vi "destroy.vi"(8 "error in":errorcluster, 11 "queue reporter in":refnum<class "queue reporter.lvclass">) -> (0 "error out":errorcluster)   [LabVIEW 2013, in "queue reporter.lvclass"]
uses:
  queue reporter.lvclass
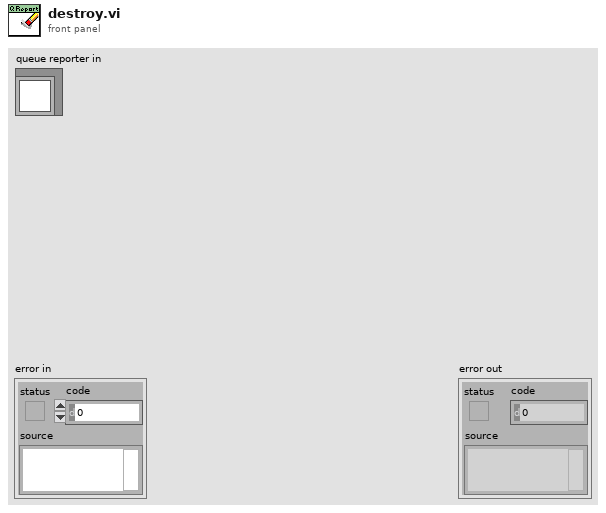
[diagram p1: front panel]
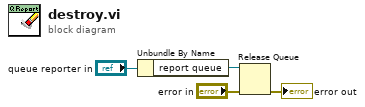
[diagram p0: block diagram]
diagram:
  n1 = Unbundle By Name("queue reporter in") -> ("report queue"=w1:refnum<queue>)
  n2 = Release Queue(queue=w1, error in (no error)="error in") -> (error out=→"error out":errorcluster)  [unwired: 1 in, 2 out]
